vi "Start Logic subvi.vi"(2 "Start":bool, 6 "Modbus master in":refnum<class "Modbus Master.lvclass">, 7 "array":string[][](array[string]), 8 "error in":errorcluster, 9 "index (row)":i32) -> (0 "Modbus master out":refnum<class "Modbus Master.lvclass">, 1 "error out":errorcluster, 3 "Time":string, 10 "Temp":string, 11 "Speed":string)   [LabVIEW 2014, in "Files Library.lvlib"]
uses:
  Files Library.lvlib
  <vilib>/NI/Modbus Library/API/Master/Modbus Master.lvclass
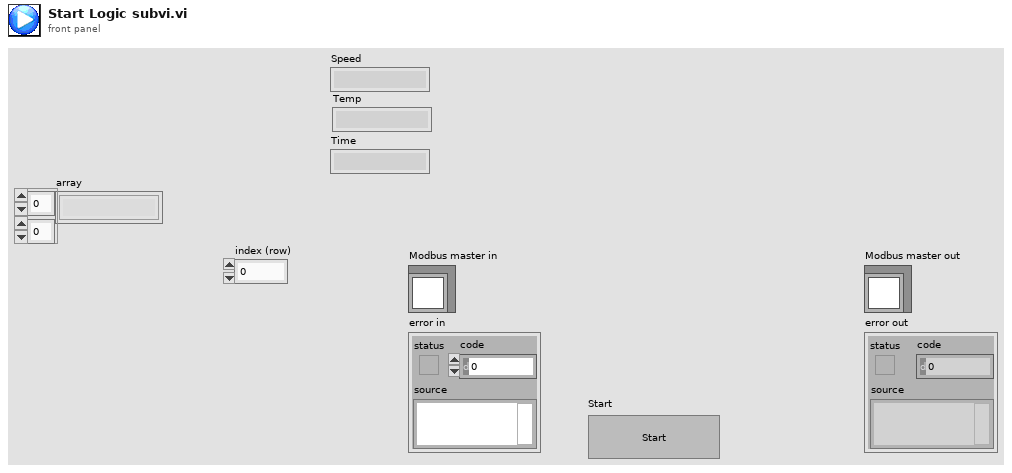
[diagram p1: front panel]
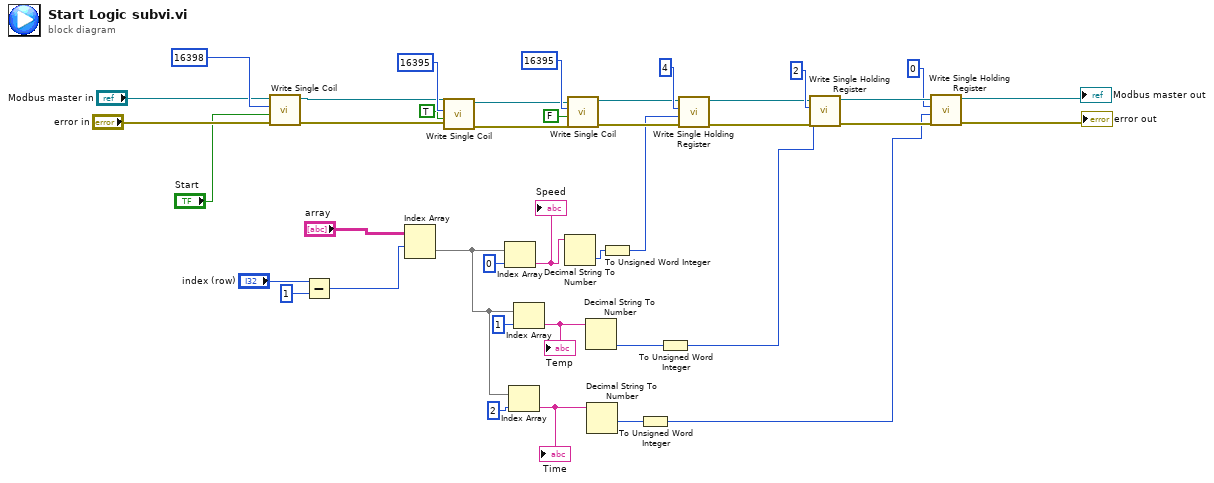
[diagram p0: block diagram]
diagram:
  n1 = call-dynamic "Write Single Coil.vi"("error in"="error in", "coil to write"="Start", "address"=u16 16398, "Modbus master in"="Modbus master in") -> ("error out"=w31:errorcluster, "Modbus master out"=w33:refnum<class "Modbus Master.lvclass">)  [unwired: 6 in]
  n2 = Subtract(x="index (row)", y=1) -> (x-y=w1:i32)
  n3 = Index Array(array="array", index (row)=w1) -> (element=w14:string[])  [unwired: 1 in]
  n4 = call-dynamic "Write Single Coil.vi"("error in"=w31, "coil to write"=TRUE, "address"=u16 16395, "Modbus master in"=w33) -> ("error out"=w30:errorcluster, "Modbus master out"=w32:refnum<class "Modbus Master.lvclass">)  [unwired: 6 in]
  n5 = Index Array(array=w14, index=0) -> (element=w15:string)
  "Speed" <- w15
  n6 = Index Array(array=w14, index=2) -> (element=w12:string)
  "Time" <- w12
  n7 = Index Array(array=w14, index=1) -> (element=w13:string)
  "Temp" <- w13
  n8 = Decimal String To Number(string=w15) -> (number=w9:i32)  [unwired: 2 in, 1 out]
  n9 = call-dynamic "Write Single Coil.vi"("error in"=w30, "coil to write"=FALSE, "address"=u16 16395, "Modbus master in"=w32) -> ("error out"=w26:errorcluster, "Modbus master out"=w27:refnum<class "Modbus Master.lvclass">)  [unwired: 6 in]
  n10 = Decimal String To Number(string=w13) -> (number=w4:i32)  [unwired: 2 in, 1 out]
  n11 = Decimal String To Number(string=w12) -> (number=w7:i32)  [unwired: 2 in, 1 out]
  n12 = To Unsigned Word Integer(number=w9) -> (unsigned 16bit integer=w8:u16)
  n13 = To Unsigned Word Integer(number=w7) -> (unsigned 16bit integer=w6:u16)
  n14 = To Unsigned Word Integer(number=w4) -> (unsigned 16bit integer=w5:u16)
  n15 = call-dynamic "Write Single Holding Register.vi"("error in"=w26, "register to write"=w8, "address"=u16 4, "Modbus master in"=w27) -> ("error out"=w24:errorcluster, "Modbus master out"=w25:refnum<class "Modbus Master.lvclass">)  [unwired: 6 in]
  n16 = call-dynamic "Write Single Holding Register.vi"("error in"=w24, "register to write"=w5, "address"=u16 2, "Modbus master in"=w25) -> ("error out"=w22:errorcluster, "Modbus master out"=w23:refnum<class "Modbus Master.lvclass">)  [unwired: 6 in]
  n17 = call-dynamic "Write Single Holding Register.vi"("error in"=w22, "register to write"=w6, "address"=u16 0, "Modbus master in"=w23) -> ("error out"=→"error out":errorcluster, "Modbus master out"=→"Modbus master out":refnum<class "Modbus Master.lvclass">)  [unwired: 6 in]
